vi "SMBUS Quick Command.vi"(7 "WriteReadFlag":u8, 9 "SlaveAddr":i16, 10 "IICIndex":i32, 11 "DevHandle":i32) -> (3 "function return":i32)   [LabVIEW 2010, in "usb2iic.lvlib"]
doc: "int WINAPI SMBUS_QuickCommand(int DevHandle,int IICIndex,short SlaveAddr,unsigned char WriteReadFlag);"
uses:
  usb2iic.lvlib
  USB2XXX.dll
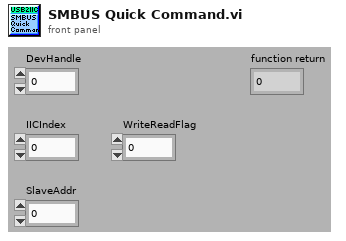
[diagram p1: front panel]
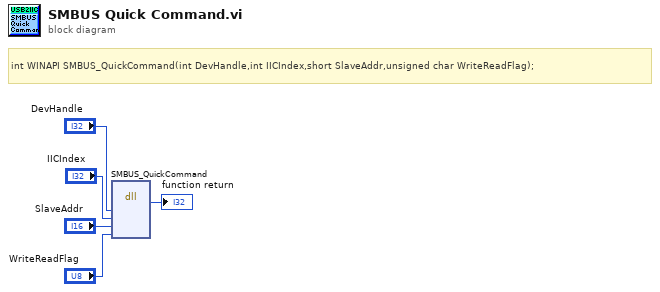
[diagram p0: block diagram]
diagram:
  # "int WINAPI SMBUS_QuickCommand(int DevHandle,int IICIndex,short SlaveAddr,unsigned char WriteReadFlag);"
  n1 = dll-call lib="G:/OtherWork/USB2XXX_Example/trunk/Labview/PublicFiles/USB2XXX.*" fn="SMBUS_QuickCommand"("DevHandle"="DevHandle", "IICIndex"="IICIndex", "SlaveAddr"="SlaveAddr", "WriteReadFlag"="WriteReadFlag") -> (→"function return":i32)  [unwired: 7 in, 2 out]
